vi "Arrange_Message.vi"(9 "Approved?":string, 10 "Average":dbl, 11 "Name":string) -> (3 "Description":string)   [LabVIEW 2025]
doc: "Arrange a message description for the student results with the provide data."
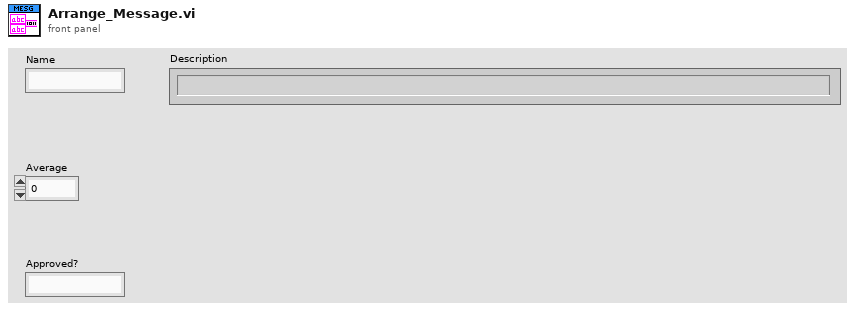
[diagram p1: front panel]
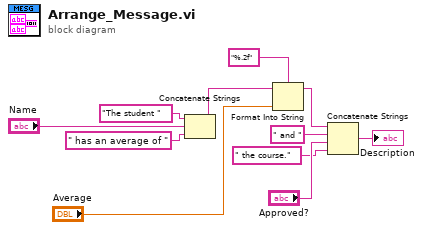
[diagram p0: block diagram]
diagram:
  n1 = Concatenate Strings("The student " ("string"), "Name", " has an average of " ("string")) -> (w4:string)
  n2 = Format Into String(format string="%.2f", initial string=w4, "Average") -> (resulting string=w6:string)  [unwired: 1 in, 1 out]
  n3 = Concatenate Strings(w6, " and " ("string"), "Approved?", " the course." ("string")) -> (→"Description":string)
